vi "Задание_АБ_рабочая_демодуляцию.vi"() -> ()   [LabVIEW 2017]
uses:
  <vilib>/Analysis/3filter.llb/Bessel Filter (DBL).vi
  <vilib>/Analysis/NI_AALBase.lvlib
panel:
  out "Итого. кол-во бит":i32
  in  "Пороговое значение":dbl
  out "Демодулированный и отфильтрованный сигнал":dbl[][](graph)
  out "Демодулированный сигнал":i16[](graph)
  in  "Нижняя частота среза":dbl
  in  "Порядок фильтра":i64(slide) scale=0.0..20.0
  in  "Переменная floor(x/y)":i32
  out "Модулирующий сигнал":dbl[](graph)
  out "Частотно модулированный цифровой сигнал":dbl[](graph)
  in  "см. 1.2 Циклов в секунду":i32(slide) scale=4.0..50.0
  in  "Сколько битов брать":i32=4
  out "Радио сигнал с паузами":dbl[](graph)
  in  "Кол-во выборок":i32=400
  out "Массив с паузами":dbl[](array[numeric])
  in  "Количество бит":i32=8
  out "Вырезка из массива":dbl[](array[numeric])
  out "Биты на выходе 1":dbl[](array[numeric])
  # "Демодуляция"
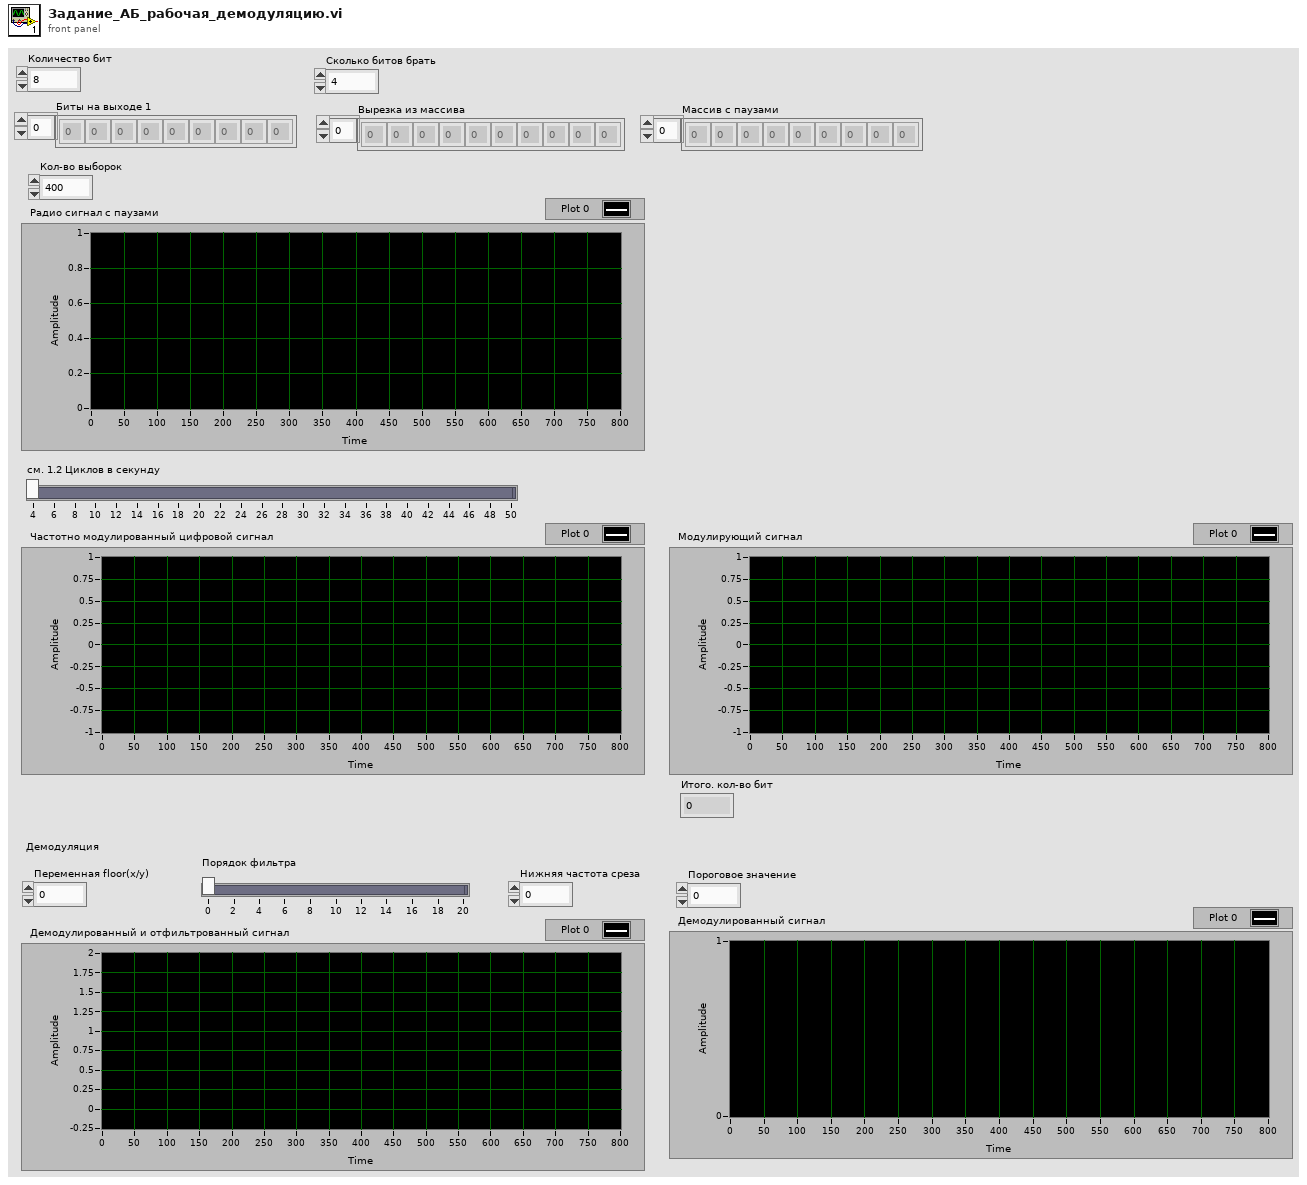
[diagram p1: front panel]
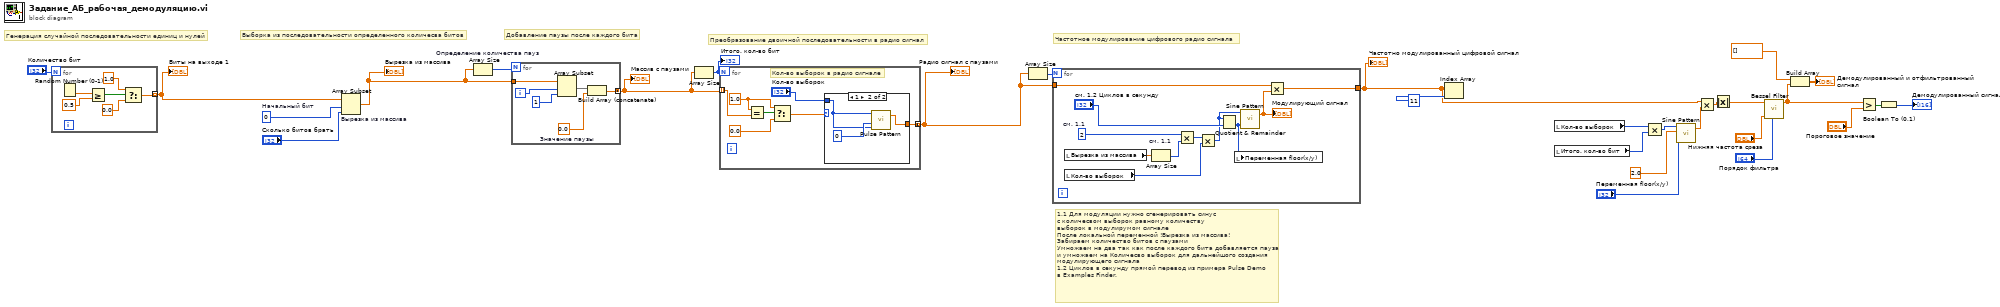
[diagram p0: block diagram]
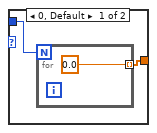
[diagram p2: hidden frame]
diagram:
  w27 = 0  # Начальный бит
  # "1.1 Для модуляции нужно сгенерировать синус \nс количесвом выборок равному количеству \nвыборок в модулирумом сигнале\nПосле локальной переменной !Вырезка из массива! \nЗабираем количество битов с паузами \nУмножаем на два так как после каждого бита добавляется пауза\nи умножаем на Количесво выборок для дальнейшого создания  \nмодулирующего сигнала\n1.2 Циклов в секунду прямой перевод из примера Pulse Demo \nв Examples Finder."
  # "Преобразование двоичной последовательности в радио сигнал"
  # "Частотное модулирование цифрового радио сигнала"
  # "Добавление паузы после каждого бита"
  # "Выборка из последовательности определенного количесва битов"
  # "Генерация случайной последовательности единиц и нулей"
  n1 = for {
    N: "Количество бит" -> [_]
    tunnel: [w29] -> w25 mode=indexing
    n2 = Random Number (0-1)() -> (number: 0 to 1=w34:dbl)
    n3 = Greater Or Equal?(x=w34, y=0.5) -> (x >= y?=w32:bool)
    n4 = Select(t=1.0, s=w32, f=0.0) -> (s? t:f=w29:dbl)
  }
  "Биты на выходе 1" <- w25
  n5 = Array Subset "Вырезка из массива"(array=w25, index=w27, length="Сколько битов брать") -> (w23:dbl[])
  "Вырезка из массива" <- w23
  n6 = Array Size "Определение количества пауз"(array=w23) -> (size(s)=w24:i32)
  n7 = for {
    N: w24 -> [_]
    tunnel: w23 -> [w37]
    tunnel: [w36] -> w20 mode=concatenating
    i -> [w35]
    w38 = 0.0  # Значение паузы
    n8 = Array Subset(array=w37, index=w35, length=1) -> (w39:dbl[])
    n9 = Build Array (concatenate)(w39, w38) -> (w36:dbl[])
  }
  "Массив с паузами" <- w20
  n10 = Array Size(array=w20) -> (size(s)=w21:i32)
  "Итого. кол-во бит" <- w21
  n11 = for {
    N: w21 -> [_]
    tunnel: w20 -> [w44] mode=indexing
    tunnel: [w42] -> w19 mode=concatenating
    w46 = 1.0
    # "Кол-во выборок в радио сигнале"
    n12 = Equal?(x=w46, y=w44) -> (x = y?=w47:bool)
    n13 = Select(t=w46, s=w47, f=0.0) -> (s? t:f=w43:dbl)
    n14 = case shown="1" w43 {
      tunnel: [w48 w52] -> w42
      tunnel: "Кол-во выборок" -> [w49 w51]
      frame 0, Default {
        n15 = for {
          N: w49 -> [_]
          tunnel: [0.0] -> w48 mode=indexing
        }
      }
      frame 1 {
        n16 = call <vilib>:"Pulse Pattern.vi"("width"=w51, "delay"=0, "samples"=w51) -> ("Pulse Pattern"=w52:dbl[])  [unwired: 1 in, 1 out]
      }
    }
  }
  "Радио сигнал с паузами" <- w19
  n17 = Array Size(array=w19) -> (size(s)=w22:i32)
  n18 = for {
    N: w22 -> [_]
    tunnel: w19 -> [w63]
    tunnel: [w62] -> w6
    w58 = 2  # см. 1.1
    n19 = local read "Вырезка из массива"() -> (w60:dbl[])
    n20 = local read "Кол-во выборок"() -> (w56:i32)
    n21 = Array Size "см. 1.1"(array=w60) -> (size(s)=w59:i32)
    n22 = Multiply(x=w58, y=w59) -> (x*y=w57:i32)
    n23 = Multiply(x=w57, y=w56) -> (x*y=w55:i32)
    n24 = Quotient & Remainder(x=w55, y="см. 1.2 Циклов в секунду") -> (floor(x/y)=w54:i32)  [unwired: 1 out]
    n25 = local write "Переменная floor(x/y)"(w54) -> ()
    n26 = call <vilib>:"Sine Pattern.vi"("cycles"=w54, "samples"=w55) -> ("Sinusoidal Pattern"=w61:dbl[])  [unwired: 2 in, 1 out]
    "Модулирующий сигнал" <- w61
    n27 = Multiply(x=w63, y=w61) -> (x*y=w62:dbl[])
  }
  "Частотно модулированный цифровой сигнал" <- w6
  n28 = Index Array(array=w6, index=11 ("index (row)")) -> ()  [unwired: 1 out]
  n29 = local read "Кол-во выборок"() -> (w2:i32)
  n30 = local read "Итого. кол-во бит"() -> (w1:i32)
  n31 = Multiply(x=w2, y=w1) -> (x*y=w3:i32)
  n32 = call <vilib>:"Sine Pattern.vi"("cycles"="Переменная floor(x/y)", "amplitude"=2.0, "samples"=w3) -> ("Sinusoidal Pattern"=w5:dbl[])  [unwired: 1 in, 1 out]
  n33 = Multiply(x=w6, y=w5) -> (x*y=w15:dbl[])
  n34 = Absolute Value(x=w15) -> (abs(x)=w12:dbl[])
  n35 = call-poly <vilib>:"Bessel Filter.vi"("order"="Порядок фильтра", "low cutoff freq: fl"="Нижняя частота среза", "X"=w12) -> ("Filtered X"=w10:dbl[])  [unwired: 5 in, 1 out]
  n36 = Build Array(dbl[] [] ("element"), w10) -> (→"Демодулированный и отфильтрованный сигнал":dbl[][])
  n37 = Greater?(x=w10, y="Пороговое значение") -> (0:w9:bool[])
  n38 = Boolean To (0,1)(Boolean=w9) -> (0, 1=→"Демодулированный сигнал":i16[])
